vi "Convert_Meters_to_Inches_Double.vi"(4 "Meters":dbl) -> (1 "Inches":dbl)   [LabVIEW 2015]
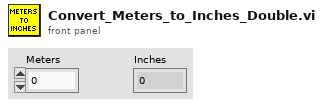
[diagram p1: front panel]
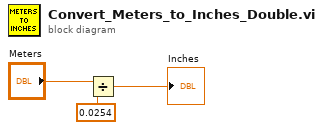
[diagram p0: block diagram]
diagram:
  n1 = Divide(x="Meters", y=0.0254) -> (x/y=→"Inches":dbl)
